vi "S-Curve Goal Calc.vi"(4 "v_f":dbl, 6 "v_i":dbl, 7 "x":dbl, 8 "t":dbl, 9 "j":dbl, 10 "a":dbl, 11 "v":dbl) -> (3 "goal":dbl)   [LabVIEW 2025]
uses:
  Trajectory/Bezier/sub-vi/Sigmoid.vi
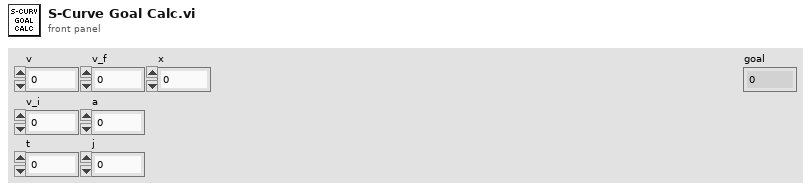
[diagram p1: front panel]
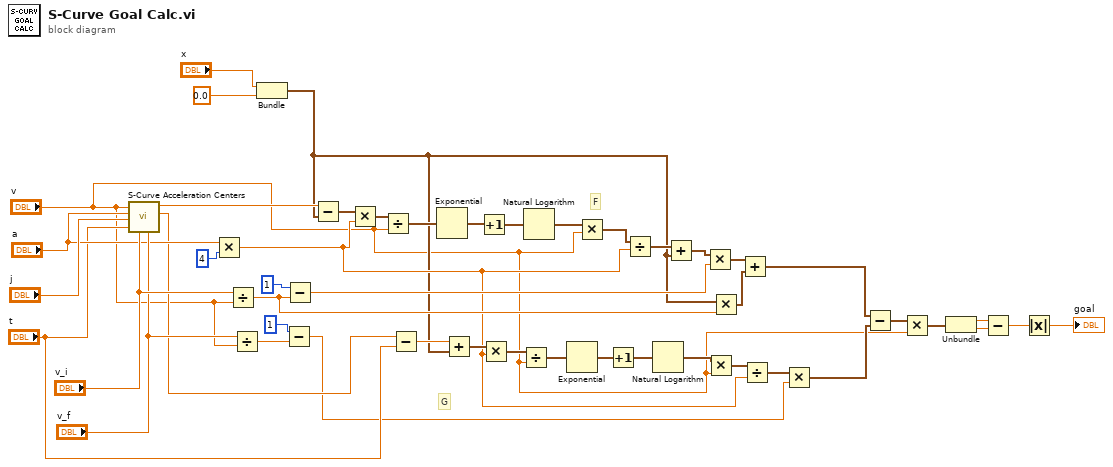
[diagram p0: block diagram]
diagram:
  # "F"
  # "G"
  n1 = call "S-Curve Acceleration Centers.vi"("v_f"="v_f", "v_i"="v_i", "t"="t", "j"="j", "a"="a", "v"="v") -> ("c2"=w25:dbl, "c1"=w39:dbl)  [unwired: 4 in]
  n2 = Multiply(x="a", y=4 ("x")) -> (x*y=w15:dbl)
  n3 = Divide(x="v_i", y="v") -> (x/y=w29:dbl)
  n4 = Divide(x="v_f", y="v") -> (x/y=w43:dbl)
  n5 = Bundle("x"="x", "x"=0.0) -> (w12:cluster{"x":dbl, "x":dbl})  [unwired: 1 in]
  n6 = Subtract(x=1, y=w43) -> (x-y=w13:dbl)
  n7 = Subtract(x=1, y=w29) -> (x-y=w31:dbl)
  n8 = Subtract(x=w39, y=w12) -> (x-y=w38:cluster{"x":dbl, "x":dbl})
  n9 = Multiply(x=w38, y=w15) -> (x*y=w37:cluster{"x":dbl, "x":dbl})
  n10 = Divide(x=w37, y="v") -> (x/y=w36:cluster{"x":dbl, "x":dbl})
  n11 = Subtract(x=w25, y="t") -> (x-y=w23:dbl)
  n12 = Exponential(1:w36) -> (0:w35:cluster{"x":dbl, "x":dbl})
  n13 = Add(x=w23, y=w12) -> (x+y=w22:cluster{"x":dbl, "x":dbl})
  n14 = Increment(x=w35) -> (x+1=w27:cluster{"x":dbl, "x":dbl})
  n15 = Multiply(x=w22, y=w15) -> (x*y=w21:cluster{"x":dbl, "x":dbl})
  n16 = Divide(x=w21, y="v") -> (x/y=w20:cluster{"x":dbl, "x":dbl})
  n17 = Natural Logarithm(1:w27) -> (0:w26:cluster{"x":dbl, "x":dbl})
  n18 = Exponential(1:w20) -> (0:w19:cluster{"x":dbl, "x":dbl})
  n19 = Multiply(x=w26, y="v") -> (x*y=w34:cluster{"x":dbl, "x":dbl})
  n20 = Increment(x=w19) -> (x+1=w18:cluster{"x":dbl, "x":dbl})
  n21 = Divide(x=w34, y=w15) -> (x/y=w33:cluster{"x":dbl, "x":dbl})
  n22 = Natural Logarithm(1:w18) -> (0:w17:cluster{"x":dbl, "x":dbl})
  n23 = Add(x=w33, y=w12) -> (x+y=w32:cluster{"x":dbl, "x":dbl})
  n24 = Multiply(x=w32, y=w31) -> (x*y=w30:cluster{"x":dbl, "x":dbl})
  n25 = Multiply(x=w17, y="v") -> (x*y=w16:cluster{"x":dbl, "x":dbl})
  n26 = Multiply(x=w12, y=w29) -> (x*y=w28:cluster{"x":dbl, "x":dbl})
  n27 = Add(x=w30, y=w28) -> (x+y=w11:cluster{"x":dbl, "x":dbl})
  n28 = Divide(x=w16, y=w15) -> (x/y=w14:cluster{"x":dbl, "x":dbl})
  n29 = Multiply(x=w14, y=w13) -> (x*y=w10:cluster{"x":dbl, "x":dbl})
  n30 = Subtract(x=w11, y=w10) -> (x-y=w9:cluster{"x":dbl, "x":dbl})
  n31 = Multiply(x=w9, y="v") -> (x*y=w7:cluster{"x":dbl, "x":dbl})
  n32 = Unbundle(w7) -> ("x"=w6:dbl, "x"=w5:dbl)
  n33 = Subtract(x=w6, y=w5) -> (x-y=w2:dbl)
  n34 = Absolute Value(x=w2) -> (abs(x)=→"goal":dbl)
